vi "Initialize Connection2.vi"(8 "error in (no error)":errorcluster, 11 "Sync Box in":refnum<class "Sync Box.lvclass">) -> (0 "error out":errorcluster, 3 "Sync Box out":refnum<class "Sync Box.lvclass">)   [LabVIEW 2018, in "Sync Box.lvclass"]
uses:
  Sync Box.lvclass
  Sync Box.lvclass/Sync Box.ctl
  Trigger/Trigger.lvclass
  StateMachine/State Machine.lvclass
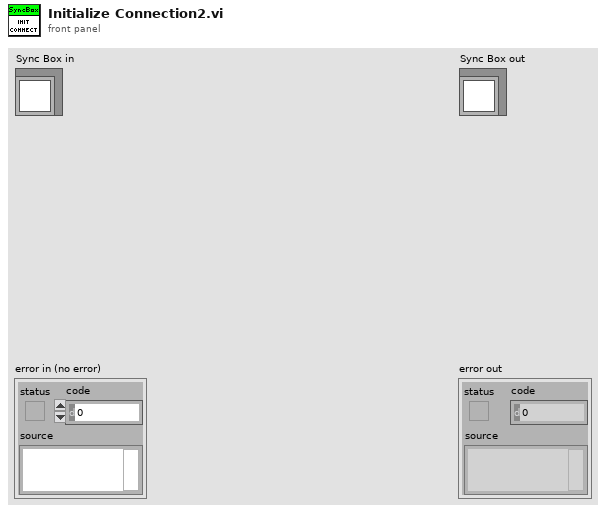
[diagram p1: front panel]
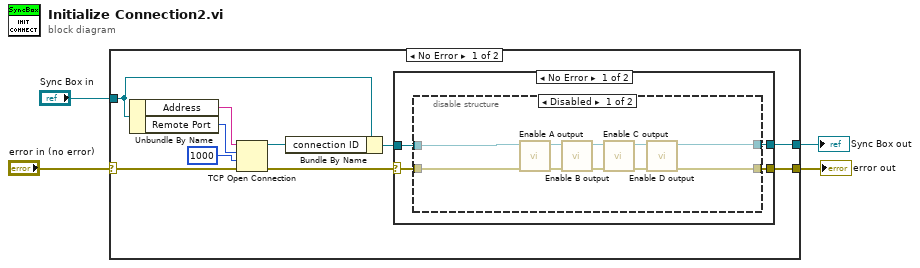
[diagram p0: block diagram]
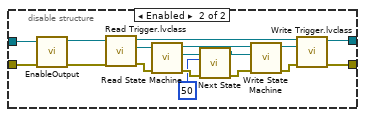
[diagram p2: hidden frame]
diagram:
  n1 = case shown="No Error" "error in (no error)" {
    selector: "error in (no error)" -> [w14 w49]
    tunnel: [w7 w49] -> w3
    tunnel: [w5 w48] -> w1
    tunnel: "Sync Box in" -> [w11 w48]
    frame No Error {
      n2 = Unbundle By Name(w11) -> ("Address"=w12:string, "Remote Port"=w13:u32)
      n3 = TCP Open Connection(address=w12, remote port or service name=w13, timeout ms (60000)=1000, error in (no error)=w14) -> (connection ID=w10:refnum<k5>, error out=w8:errorcluster)  [unwired: 1 in]
      n4 = Bundle By Name(cluster=w11, "connection ID"=w10) -> (w6:refnum<class "Sync Box.lvclass">)
      n5 = case shown="No Error" w8 {
        selector: w8 -> [w18 w46]
        tunnel: [w17 w46] -> w7
        tunnel: w6 -> [w16 w47]
        tunnel: [w15 w47] -> w5
        frame No Error {
          n6 = disable-structure shown="Disabled" {
            disable-tunnel: w18 -> [w22 w44]
            disable-tunnel: [w21 w33] -> w17
            disable-tunnel: w16 -> [w20 w45]
            disable-tunnel: [w19 w32] -> w15
            frame Disabled {
              n7 = call "Enable A output.vi"("error in (no error)"=w22, "Sync Box in"=w20) -> ("error out"=w28:errorcluster, "Sync Box out"=w23:refnum<class "Sync Box.lvclass">)  [unwired: 8 in]
              n8 = call "Enable B output.vi"("error in (no error)"=w28, "Sync Box in"=w23) -> ("error out"=w27:errorcluster, "Sync Box out"=w24:refnum<class "Sync Box.lvclass">)  [unwired: 8 in]
              n9 = call "Enable C output.vi"("error in (no error)"=w27, "Sync Box in"=w24) -> ("error out"=w26:errorcluster, "Sync Box out"=w25:refnum<class "Sync Box.lvclass">)  [unwired: 8 in]
              n10 = call "Enable D output.vi"("error in (no error)"=w26, "Sync Box in"=w25) -> ("error out"=w21:errorcluster, "Sync Box out"=w19:refnum<class "Sync Box.lvclass">)  [unwired: 8 in]
            }
            frame Enabled {
              n11 = call-dynamic "EnableOutput.vi"("error in (no error)"=w44, "Sync Box in"=w45) -> ("error out"=w38:errorcluster, "Sync Box out"=w43:refnum<class "Sync Box.lvclass">)  [unwired: 8 in]
              n12 = call-dynamic "Read Trigger.lvclass.vi"("error in (no error)"=w38, "Sync Box in"=w43) -> ("error out"=w37:errorcluster, "Trigger.lvclass"=w41:refnum<class "Trigger.lvclass">, "Sync Box out"=w42:refnum<class "Sync Box.lvclass">)  [unwired: 7 in]
              n13 = call-dynamic "Read State Machine.vi"("error in (no error)"=w37, "Device in"=w41) -> ("error out"=w36:errorcluster, "State Machine.lvclass"=w31:refnum<class "State Machine.lvclass">, "Device out"=w40:refnum<class "Trigger.lvclass">)  [unwired: 7 in]
              n14 = call "Next State.vi"("error in (no error)"=w36, "New_State"=u32 50, "State Machine in"=w31) -> ("error out"=w35:errorcluster, "State Machine out"=w30:refnum<class "State Machine.lvclass">)  [unwired: 7 in]
              n15 = call-dynamic "Write State Machine.vi"("error in (no error)"=w35, "State Machine.lvclass"=w30, "Device in"=w40) -> ("error out"=w34:errorcluster, "Device out"=w39:refnum<class "Trigger.lvclass">)  [unwired: 7 in]
              n16 = call-dynamic "Write Trigger.lvclass.vi"("error in (no error)"=w34, "Trigger.lvclass"=w39, "Sync Box in"=w42) -> ("error out"=w33:errorcluster, "Sync Box out"=w32:refnum<class "Sync Box.lvclass">)  [unwired: 7 in]
            }
          }
        }
        frame Error {
        }
      }
    }
    frame Error {
    }
  }
  "error out" <- w3
  "Sync Box out" <- w1
